vi "Happen YAML.vi"(4 "Condensed?":bool, 6 "No Label?":bool, 8 "error in (no error)":errorcluster, 9 "Level":u32, 10 "Anything":variant, 11 "YAML String in":string) -> (0 "error out":errorcluster, 3 "YAML String out":string)   [LabVIEW 2015, in "YAML Parser.lvlib"]
uses:
  YAML Parser.lvlib
  <vilib>/Utility/Data Type/Type Definitions/Data Type.ctl
  <vilib>/ErrorRing/Error Ring.xnode
  <vilib>/Utility/Data Type/NI_Data Type.lvlib
  <vilib>/Utility/error.llb/whitespace.ctl
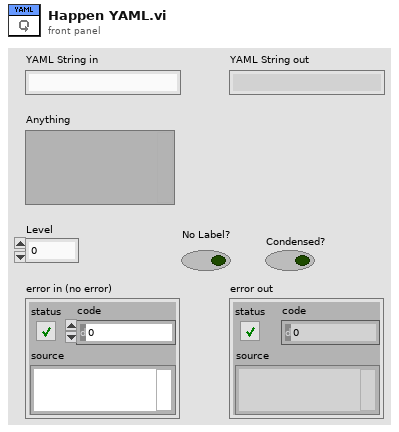
[diagram p1: front panel]
types:
  T1 = typedef "NI_Data Type.lvlib/Data Type.ctl" = enum8{"Invalid Type", "Void", "I8", "I16", "I32", "I64", "U8", "U16", "U32", "U64", "Single Float", "Double Float", "Extended Float", "Single Complex", "Double Complex", "Extended Complex", "Enum U8", "Enum U16", "Enum U32", "Enum U64", "Single Float With Unit", "Double Float With Unit", "Extended Float With Unit", "Single Complex with Unit", "Double Complex with Unit", "Extended Complex with Unit", "Boolean", "String", "Path", "Picture", "Tag", "Array", "Cluster", "Variant", "LV Variant", "Waveform", "Timestamp", "Digital Waveform", "Digital Data", "ExpressData", "Refnum", "External Data", "VI", "Poly VI", "LabVIEW Class Instance", "Fixed Point"}
  T2 = typedef "whitespace.ctl" = u16
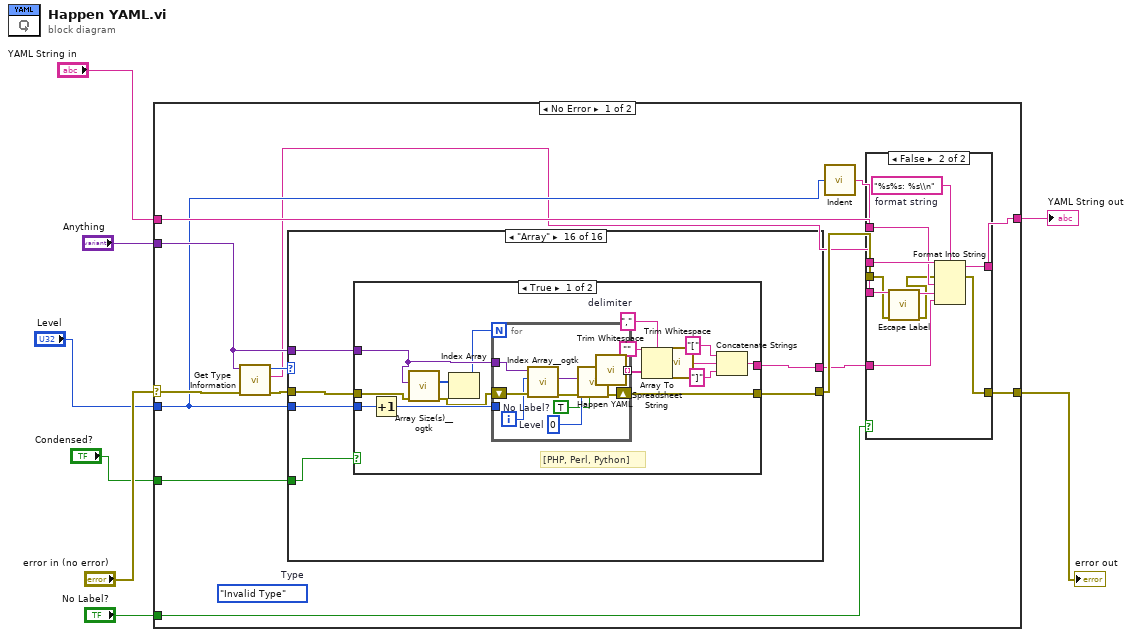
[diagram p0: block diagram]
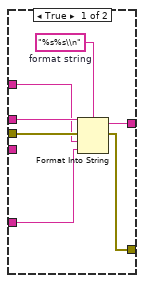
[diagram p2: hidden frame]
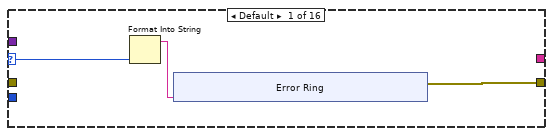
[diagram p3: hidden frame]
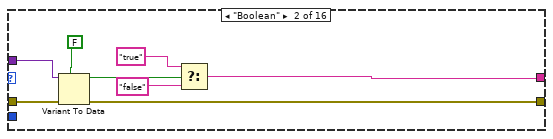
[diagram p4: hidden frame]
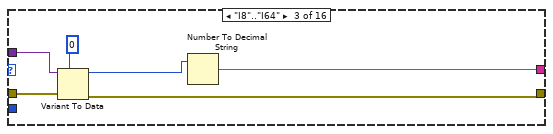
[diagram p5: hidden frame]
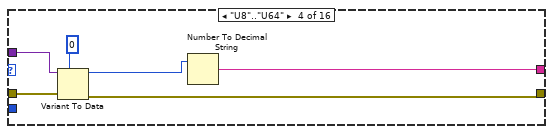
[diagram p6: hidden frame]
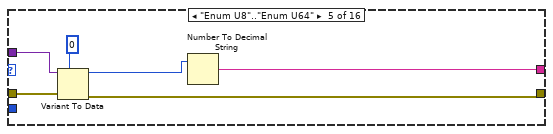
[diagram p7: hidden frame]
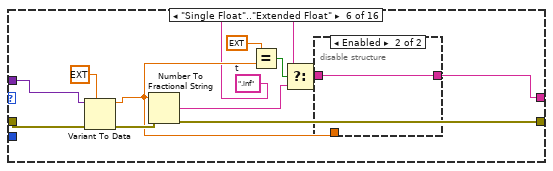
[diagram p8: hidden frame]
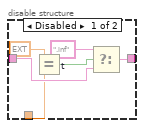
[diagram p9: hidden frame]
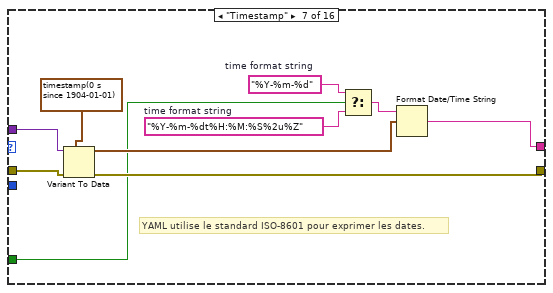
[diagram p10: hidden frame]
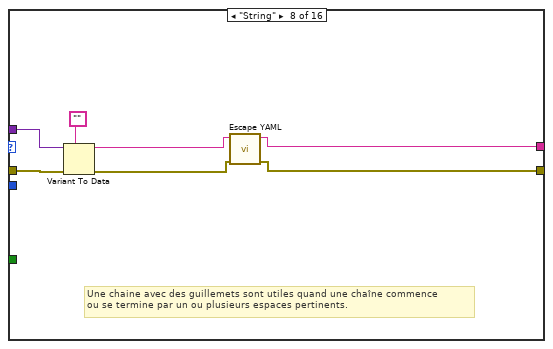
[diagram p11: hidden frame]
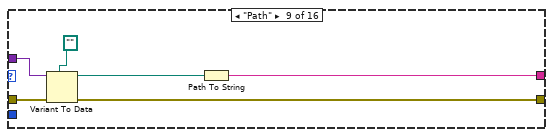
[diagram p12: hidden frame]
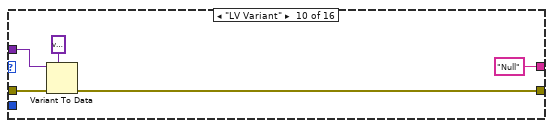
[diagram p13: hidden frame]
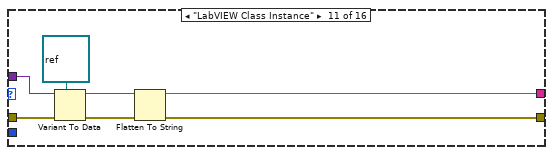
[diagram p14: hidden frame]
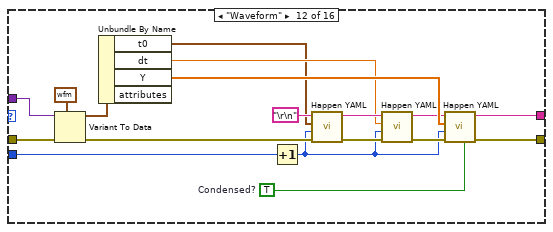
[diagram p15: hidden frame]
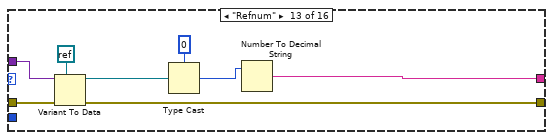
[diagram p16: hidden frame]
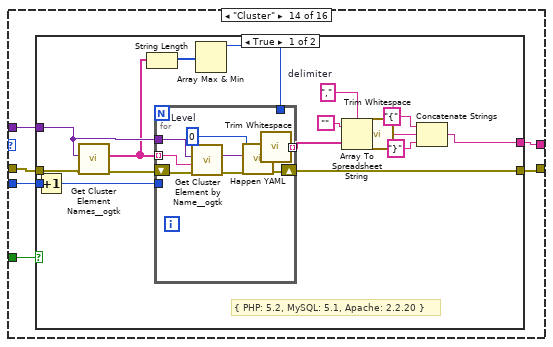
[diagram p17: hidden frame]
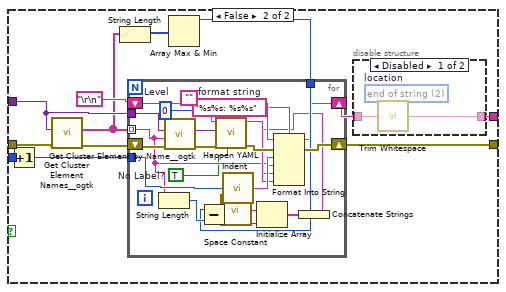
[diagram p18: hidden frame]
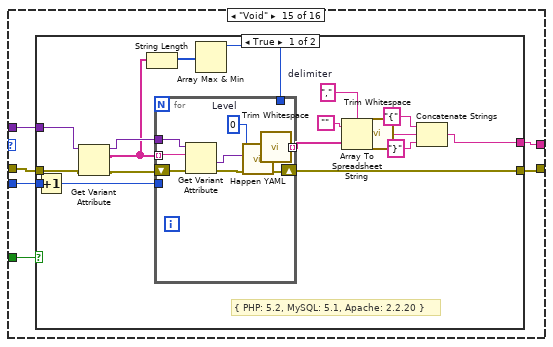
[diagram p20: hidden frame]
diagram:
  n1 = case shown="No Error" "error in (no error)" {
    selector: "error in (no error)" -> [w22 w351]
    tunnel: [w17 w351] -> w7
    tunnel: "Anything" -> [w19 _]
    tunnel: [w15 _] -> w5
    tunnel: "Level" -> [w13 _]
    tunnel: "YAML String in" -> [w14 _]
    tunnel: "No Label?" -> [w11 _]
    tunnel: "Condensed?" -> [w10 _]
    frame No Error {
      (unwired) Data_Type."Invalid Type"  # Type
      n2 = call <vilib>:"Get Type Information.vi"("error in (no error)"=w22, "Variant"=w19) -> ("error out"=w20:errorcluster, "Name"=w9:string, "Type"=w21:T1)  [unwired: 5 in, 2 out]
      n3 = case shown="\"Array\"" w21 {
        selector: w21 -> [w41 _ _ _ _ _ _ _ _ _ _ _ _ _ _ _]
        tunnel: w20 -> [_ w55 w61 w67 w73 w84 w101 w107 w114 w119 w126 w144 w152 w156 w226 w296]
        tunnel: w19 -> [_ w54 w60 w66 w72 w83 w100 w106 w113 w118 w125 w143 w151 w155 w225 w295]
        tunnel: [w42 w52 w58 w64 w70 w81 w97 w103 w109 w117 w122 w139 w150 w158 w228 w299] -> w18
        tunnel: [_ w48 w56 w62 w68 w74 w96 w102 w110 "Null" w120 w138 w145 w154 w224 w298] -> w16
        tunnel: w13 -> [_ _ _ _ _ _ _ _ _ _ _ w137 _ w157 w227 w297]
        tunnel: w10 -> [_ _ _ _ _ _ w95 _ _ _ _ _ _ w153 w223 w294]
        frame Default {
          n4 = Format Into String(w41) -> (resulting string=w40:string)  [unwired: 3 in, 1 out]
          n5 = xnode "Error Ring"("parameter 0"=w40) -> ("error out"=w42:errorcluster)
        }
        frame "Boolean" {
          n6 = Variant To Data(error in=w55, type=FALSE, Variant=w54) -> (data=w51:bool, error out=w52:errorcluster)
          n7 = Select(t="true", s=w51, f="false") -> (s? t:f=w48:string)
        }
        frame "I8".."I64" {
          n8 = Variant To Data(error in=w61, type=i64 0, Variant=w60) -> (data=w57:i64, error out=w58:errorcluster)
          n9 = Number To Decimal String(number=w57) -> (decimal integer string=w56:string)  [unwired: 1 in]
        }
        frame "U8".."U64" {
          n10 = Variant To Data(error in=w67, type=u64 0, Variant=w66) -> (data=w63:u64, error out=w64:errorcluster)
          n11 = Number To Decimal String(number=w63) -> (decimal integer string=w62:string)  [unwired: 1 in]
        }
        frame "Enum U8".."Enum U64" {
          n12 = Variant To Data(error in=w73, type=u64 0, Variant=w72) -> (data=w69:u64, error out=w70:errorcluster)
          n13 = Number To Decimal String(number=w69) -> (decimal integer string=w68:string)  [unwired: 1 in]
        }
        frame "Single Float".."Extended Float" {
          w75 = ".inf"  # t
          n14 = Variant To Data(error in=w84, type=ext 0.0, Variant=w83) -> (data=w76:ext, error out=w81:errorcluster)
          n15 = Number To Fractional String(number=w76) -> (F-format string=w78:string)  [unwired: 3 in]
          n16 = Equal?(x=ext inf, y=w76) -> (x = y?=w79:bool)
          n17 = Select(t=w75, s=w79, f=w78) -> (s? t:f=w77:string)
          n18 = disable-structure shown="Enabled" {
            disable-tunnel: w77 -> [w88 w91]
            disable-tunnel: w76 -> [w87 _]
            disable-tunnel: [w85 w91] -> w74
            frame Disabled {
              w86 = ".inf"  # t
              n19 = Equal?(x=ext -inf, y=w87) -> (x = y?=w89:bool)
              n20 = Select(t=w86, s=w89, f=w88) -> (s? t:f=w85:string)
            }
            frame Enabled {
            }
          }
        }
        frame "Timestamp" {
          w93 = "%Y-%m-%d"  # time format string
          w94 = "%Y-%m-%dt%H:%M:%S%2u%Z"  # time format string
          # "YAML utilise le standard ISO-8601 pour exprimer les dates."
          n21 = Variant To Data(error in=w101, type=timestamp(0 s since 1904-01-01), Variant=w100) -> (data=w98:timestamp, error out=w97:errorcluster)
          n22 = Select(t=w93, s=w95, f=w94) -> (s? t:f=w92:string)
          n23 = Format Date/Time String(time format string (%c)=w92, seconds (now)=w98) -> (date/time string=w96:string)  [unwired: 1 in]
        }
        frame "String" {
          # "Une chaine avec des guillemets sont utiles quand une chaîne commence \nou se termine par un ou plusieurs espaces pertinents."
          n24 = Variant To Data(error in=w107, type="", Variant=w106) -> (data=w105:string, error out=w104:errorcluster)
          n25 = call "Escape YAML.vi"("error in (no error)"=w104, "String"=w105) -> ("error out"=w103:errorcluster, "YAML String"=w102:string)  [unwired: 8 in]
        }
        frame "Path" {
          n26 = Variant To Data(error in=w114, type=path "", Variant=w113) -> (data=w111:path, error out=w109:errorcluster)
          n27 = Path To String(path=w111) -> (string=w110:string)
        }
        frame "LV Variant" {
          n28 = Variant To Data(error in=w119, type=variant, Variant=w118) -> (error out=w117:errorcluster)  [unwired: 1 out]
        }
        frame "LabVIEW Class Instance" {
          n29 = Variant To Data(error in=w126, type=refnum<class> refnum, Variant=w125) -> (data=w121:refnum<class>, error out=w123:errorcluster)
          n30 = Flatten To String(anything=w121, error in (no error)=w123) -> (data string=w120:string, error out=w122:errorcluster)  [unwired: 2 in, 1 out]
        }
        frame "Waveform" {
          w127 = TRUE  # Condensed?
          n31 = Variant To Data(error in=w144, type=waveform(dbl) {"t0"=timestamp(0 s since 1904-01-01), "dt"=1.0, "Y"=[]}, Variant=w143) -> (data=w141:waveform(dbl), error out=w140:errorcluster)
          n32 = Unbundle By Name(w141) -> ("t0"=w128:timestamp, "dt"=w130:dbl, "Y"=w133:dbl[])  [unwired: 1 out]
          n33 = Increment(x=w137) -> (x+1=w134:u32)
          n34 = call "Happen YAML.vi"("error in (no error)"=w140, "Level"=w134, "Anything"=w128, "YAML String in"="\r\n") -> ("error out"=w136:errorcluster, "YAML String out"=w131:string)  [unwired: 6 in]
          n35 = call "Happen YAML.vi"("error in (no error)"=w136, "Level"=w134, "Anything"=w130, "YAML String in"=w131) -> ("error out"=w135:errorcluster, "YAML String out"=w132:string)  [unwired: 6 in]
          n36 = call "Happen YAML.vi"("Condensed?"=w127, "error in (no error)"=w135, "Level"=w134, "Anything"=w133, "YAML String in"=w132) -> ("error out"=w139:errorcluster, "YAML String out"=w138:string)  [unwired: 5 in]
        }
        frame "Refnum" {
          n37 = Variant To Data(error in=w152, type=refnum<k0> refnum, Variant=w151) -> (data=w147:refnum<k0>, error out=w150:errorcluster)
          n38 = Type Cast(type=u32 0, x=w147) -> (*(type *) &x=w146:u32)
          n39 = Number To Decimal String(number=w146) -> (decimal integer string=w145:string)  [unwired: 1 in]
        }
        frame "Cluster" {
          n40 = case shown="True" w153 {
            tunnel: [w175 w196] -> w158
            tunnel: w157 -> [w174 w193]
            tunnel: w156 -> [w172 w191]
            tunnel: w155 -> [w170 w189]
            tunnel: [w160 w188] -> w154
            frame True {
              w166 = ","  # delimiter
              # "{ PHP: 5.2, MySQL: 5.1, Apache: 2.2.20 }"
              n41 = Increment(x=w174) -> (x+1=w173:u32)
              n42 = call <userlib>:"Get Cluster Element Names__ogtk.vi"("error in (no error)"=w172, "Cluster"=w170) -> ("error out"=w171:errorcluster, "Element Names"=w169:string[])  [unwired: 8 in]
              n43 = String Length(string=w169) -> (length=w168:i32[])
              n44 = Array Max & Min(array=w168) -> (max value=w167:i32)  [unwired: 3 out]
              n45 = for {
                shift-right: [w178] -> w175
                shift-left: w171 -> [w184]
                tunnel: w173 -> [_]
                tunnel: w169 -> [w181] mode=indexing
                tunnel: w170 -> [w183]
                tunnel: w167 -> [_]
                tunnel: [w177] -> w162 mode=indexing
                w180 = u32 0  # Level
                n46 = call <userlib>:"Get Cluster Element by Name__ogtk.vi"("error in (no error)"=w184, "Element Name"=w181, "Cluster"=w183) -> ("error out"=w182:errorcluster, "VElement"=w176:variant)  [unwired: 6 in, 1 out]
                n47 = call "Happen YAML.vi"("error in (no error)"=w182, "Level"=w180, "Anything"=w176) -> ("error out"=w178:errorcluster, "YAML String out"=w179:string)  [unwired: 7 in]
                n48 = call <vilib>:"Trim Whitespace.vi"("string"=w179) -> ("trimmed string"=w177:string)  [unwired: 1 in]
              }
              n49 = Array To Spreadsheet String(delimiter (Tab)=w166, array=w162, 3:"") -> (spreadsheet string=w165:string)
              n50 = call <vilib>:"Trim Whitespace.vi"("string"=w165) -> ("trimmed string"=w159:string)  [unwired: 1 in]
              n51 = Concatenate Strings("{", w159, "}") -> (w160:string)
            }
            frame False {
              n52 = Increment(x=w193) -> (x+1=w192:u32)
              n53 = call <userlib>:"Get Cluster Element Names__ogtk.vi"("error in (no error)"=w191, "Cluster"=w189) -> ("error out"=w190:errorcluster, "Element Names"=w187:string[])  [unwired: 8 in]
              n54 = String Length(string=w187) -> (length=w186:i32[])
              n55 = Array Max & Min(array=w186) -> (max value=w185:i32)  [unwired: 3 out]
              n56 = for {
                shift-right: [w218] -> w196
                shift-left: w190 -> [w222]
                shift-right: [w205] -> w194
                shift-left: "\r\n" -> [w217]
                tunnel: w192 -> [w216]
                tunnel: w187 -> [w212] mode=indexing
                tunnel: w189 -> [w221]
                tunnel: w185 -> [w210]
                w204 = u32 0  # Level
                w215 = "%s%s: %s%s"  # format string
                w201 = TRUE  # No Label?
                n57 = String Length(string=w212) -> (length=w211:i32)
                n58 = call <userlib>:"Get Cluster Element by Name__ogtk.vi"("error in (no error)"=w222, "Element Name"=w212, "Cluster"=w221) -> ("error out"=w220:errorcluster, "VElement"=w202:variant)  [unwired: 6 in, 1 out]
                n59 = Subtract(x=w210, y=w211) -> (x-y=w207:i32)
                n60 = call "Happen YAML.vi"("No Label?"=w201, "error in (no error)"=w220, "Level"=w204, "Anything"=w202, "YAML String in"="") -> ("error out"=w219:errorcluster, "YAML String out"=w213:string)  [unwired: 5 in]
                n61 = call <vilib>:"Space Constant.vi"() -> ("String"=w209:string)
                n62 = call "Indent.vi"("Index"=w216) -> ("Indentation"=w214:string)
                n63 = Initialize Array(w209, w207) -> (w208:string[])
                n64 = Concatenate Strings(w208) -> (w206:string)
                n65 = Format Into String(format string=w215, initial string=w217, error in=w219, w214, w212, w206, w213) -> (resulting string=w205:string, error out=w218:errorcluster)
              }
              n66 = disable-structure shown="Disabled" {
                disable-tunnel: w194 -> [w199 w200]
                disable-tunnel: [w198 w200] -> w188
                frame Disabled {
                  w197 = T2 2 items=["both", "start of string", "end of string"]  # location
                  n67 = call <vilib>:"Trim Whitespace.vi"("string"=w199, "location (both)"=w197) -> ("trimmed string"=w198:string)
                }
                frame Enabled {
                }
              }
            }
          }
        }
        frame "Void" {
          n68 = case shown="True" w223 {
            tunnel: [w246 w268] -> w228
            tunnel: w227 -> [w245 w265]
            tunnel: w226 -> [w233 w260]
            tunnel: w225 -> [w232 w257]
            tunnel: [w235 w263] -> w224
            frame True {
              w241 = ","  # delimiter
              # "{ PHP: 5.2, MySQL: 5.1, Apache: 2.2.20 }"
              n69 = Increment(x=w245) -> (x+1=w244:u32)
              n70 = Get Variant Attribute(Variant=w232, error in=w233) -> (duplicate Variant=w231:variant, names=w230:string[], error out=w229:errorcluster)  [unwired: 2 in, 1 out]
              n71 = String Length(string=w230) -> (length=w243:i32[])
              n72 = Array Max & Min(array=w243) -> (max value=w242:i32)  [unwired: 3 out]
              n73 = for {
                shift-right: [w253] -> w246
                shift-left: w229 -> [w251]
                tunnel: w244 -> [_]
                tunnel: w230 -> [w250] mode=indexing
                tunnel: w231 -> [w249]
                tunnel: w242 -> [_]
                tunnel: [w252] -> w237 mode=indexing
                w255 = u32 0  # Level
                n74 = Get Variant Attribute(Variant=w249, name=w250, error in=w251) -> (value=w247:variant, error out=w248:errorcluster)  [unwired: 1 in, 2 out]
                n75 = call "Happen YAML.vi"("error in (no error)"=w248, "Level"=w255, "Anything"=w247) -> ("error out"=w253:errorcluster, "YAML String out"=w254:string)  [unwired: 7 in]
                n76 = call <vilib>:"Trim Whitespace.vi"("string"=w254) -> ("trimmed string"=w252:string)  [unwired: 1 in]
              }
              n77 = Array To Spreadsheet String(delimiter (Tab)=w241, array=w237, 3:"") -> (spreadsheet string=w240:string)
              n78 = call <vilib>:"Trim Whitespace.vi"("string"=w240) -> ("trimmed string"=w234:string)  [unwired: 1 in]
              n79 = Concatenate Strings("{", w234, "}") -> (w235:string)
            }
            frame False {
              n80 = Increment(x=w265) -> (x+1=w264:u32)
              n81 = Get Variant Attribute(Variant=w257, error in=w260) -> (duplicate Variant=w256:variant, names=w258:string[], error out=w259:errorcluster)  [unwired: 2 in, 1 out]
              n82 = String Length(string=w258) -> (length=w262:i32[])
              n83 = Array Max & Min(array=w262) -> (max value=w261:i32)  [unwired: 3 out]
              n84 = for {
                shift-right: [w292] -> w268
                shift-left: w259 -> [w278]
                shift-right: [w281] -> w266
                shift-left: "\r\n" -> [w291]
                tunnel: w264 -> [w276]
                tunnel: w258 -> [w279] mode=indexing
                tunnel: w261 -> [w286]
                tunnel: w256 -> [w280]
                w290 = "%s%s: %s%s"  # format string
                w273 = TRUE  # No Label?
                n85 = Get Variant Attribute(Variant=w280, name=w279, error in=w278) -> (value=w274:variant, error out=w277:errorcluster)  [unwired: 1 in, 2 out]
                n86 = String Length(string=w279) -> (length=w287:i32)
                n87 = Subtract(x=w286, y=w287) -> (x-y=w283:i32)
                n88 = call "Happen YAML.vi"("No Label?"=w273, "error in (no error)"=w277, "Level"=w276, "Anything"=w274, "YAML String in"="") -> ("error out"=w293:errorcluster, "YAML String out"=w288:string)  [unwired: 5 in]
                n89 = call <vilib>:"Space Constant.vi"() -> ("String"=w285:string)
                n90 = call "Indent.vi"("Index"=w276) -> ("Indentation"=w289:string)
                n91 = Initialize Array(w285, w283) -> (w284:string[])
                n92 = Concatenate Strings(w284) -> (w282:string)
                n93 = Format Into String(format string=w290, initial string=w291, error in=w293, w289, w279, w282, w288) -> (resulting string=w281:string, error out=w292:errorcluster)
              }
              n94 = disable-structure shown="Disabled" {
                disable-tunnel: w266 -> [w271 w272]
                disable-tunnel: [w270 w272] -> w263
                frame Disabled {
                  w269 = T2 2 items=["both", "start of string", "end of string"]  # location
                  n95 = call <vilib>:"Trim Whitespace.vi"("string"=w271, "location (both)"=w269) -> ("trimmed string"=w270:string)
                }
                frame Enabled {
                }
              }
            }
          }
        }
        frame "Array" {
          n96 = case shown="True" w294 {
            tunnel: [w315 w335] -> w299
            tunnel: [w304 w333] -> w298
            tunnel: w297 -> [w314 w332]
            tunnel: w296 -> [w312 w330]
            tunnel: w295 -> [w311 w329]
            frame True {
              w306 = ","  # delimiter
              # "[PHP, Perl, Python]"
              n97 = Increment(x=w314) -> (x+1=w313:u32)
              n98 = call <userlib>:"Array Size(s)__ogtk.vi"("error in (no error)"=w312, "Array"=w311) -> ("error out"=w308:errorcluster, "Size(s)"=w310:u32[])  [unwired: 7 in, 1 out]
              n99 = Index Array(array=w310) -> (element=w309:u32)  [unwired: 1 in]
              n100 = for {
                N: w309 -> [_]
                shift-right: [w320] -> w315
                shift-left: w308 -> [w325]
                tunnel: w313 -> [_]
                tunnel: w311 -> [w324]
                tunnel: [w318] -> w307 mode=indexing
                i -> [w322]
                w316 = TRUE  # No Label?
                w321 = u32 0  # Level
                n101 = call <userlib>:"Index Array__ogtk.vi"("error in (no error)"=w325, "Index (1D)"=w322, "MultiD Array"=w324) -> ("error out"=w323:errorcluster, "Array Element"=w317:variant)  [unwired: 7 in]
                n102 = call "Happen YAML.vi"("No Label?"=w316, "error in (no error)"=w323, "Level"=w321, "Anything"=w317) -> ("error out"=w320:errorcluster, "YAML String out"=w319:string)  [unwired: 6 in]
                n103 = call <vilib>:"Trim Whitespace.vi"("string"=w319) -> ("trimmed string"=w318:string)  [unwired: 1 in]
              }
              n104 = Array To Spreadsheet String(delimiter (Tab)=w306, array=w307, 3:"") -> (spreadsheet string=w305:string)
              n105 = call <vilib>:"Trim Whitespace.vi"("string"=w305) -> ("trimmed string"=w300:string)  [unwired: 1 in]
              n106 = Concatenate Strings("[", w300, "]") -> (w304:string)
            }
            frame False {
              n107 = Increment(x=w332) -> (x+1=w331:u32)
              n108 = call <userlib>:"Array Size(s)__ogtk.vi"("error in (no error)"=w330, "Array"=w329) -> ("error out"=w326:errorcluster, "Size(s)"=w328:u32[])  [unwired: 7 in, 1 out]
              n109 = Index Array(array=w328) -> (element=w327:u32)  [unwired: 1 in]
              n110 = for {
                N: w327 -> [_]
                shift-right: [w345] -> w335
                shift-left: w326 -> [w350]
                shift-right: [w339] -> w333
                shift-left: "\r\n" -> [w344]
                tunnel: w331 -> [w342]
                tunnel: w329 -> [w349]
                i -> [w347]
                w336 = TRUE  # No Label?
                w338 = u32 0  # Level
                w343 = "%s- %s"  # format string
                n111 = call <userlib>:"Index Array__ogtk.vi"("error in (no error)"=w350, "Index (1D)"=w347, "MultiD Array"=w349) -> ("error out"=w348:errorcluster, "Array Element"=w337:variant)  [unwired: 7 in]
                n112 = call "Happen YAML.vi"("No Label?"=w336, "error in (no error)"=w348, "Level"=w338, "Anything"=w337) -> ("error out"=w346:errorcluster, "YAML String out"=w340:string)  [unwired: 6 in]
                n113 = call "Indent.vi"("Index"=w342) -> ("Indentation"=w341:string)
                n114 = Format Into String(format string=w343, initial string=w344, error in=w346, w341, w340) -> (resulting string=w339:string, error out=w345:errorcluster)
              }
            }
          }
        }
      }
      n115 = call "Indent.vi"("Index"=w13) -> ("Indentation"=w12:string)
      n116 = case shown="False" w11 {
        tunnel: w9 -> [_ w33]
        tunnel: w18 -> [w28 w31]
        tunnel: [w27 w38] -> w17
        tunnel: w16 -> [w26 w37]
        tunnel: [w25 w36] -> w15
        tunnel: w14 -> [w24 w35]
        tunnel: w12 -> [w23 w34]
        frame True {
          w29 = "%s%s\\n"  # format string
          n117 = Format Into String(format string=w29, initial string=w24, error in=w28, w23, w26) -> (resulting string=w25:string, error out=w27:errorcluster)
        }
        frame False {
          w39 = "%s%s: %s\\n"  # format string
          n118 = call "Escape Label.vi"("error in (no error)"=w31, "Label"=w33) -> ("error out"=w30:errorcluster, "YAML Label"=w32:string)  [unwired: 8 in]
          n119 = Format Into String(format string=w39, initial string=w35, error in=w30, w34, w32, w37) -> (resulting string=w36:string, error out=w38:errorcluster)
        }
      }
    }
    frame Error {
    }
  }
  "error out" <- w7
  "YAML String out" <- w5
